vi "CREATE CHECK IN QUERY.vi"(0 "What to Search":string, 5 "Search Column Name":string, 7 "Sorting Column Name":string, 9 "Column to Search In":u16, 11 "Column to Sort By":u16, 12 "Date Range":u16(ring) items=["Greater Than", "Less Than", "Between"], 13 "Dates Less Than":string="8/1/2023", 14 "Dates Greater Than":string="8/1/2023") -> (4 "SQL QUERY":string)   [LabVIEW 2019]
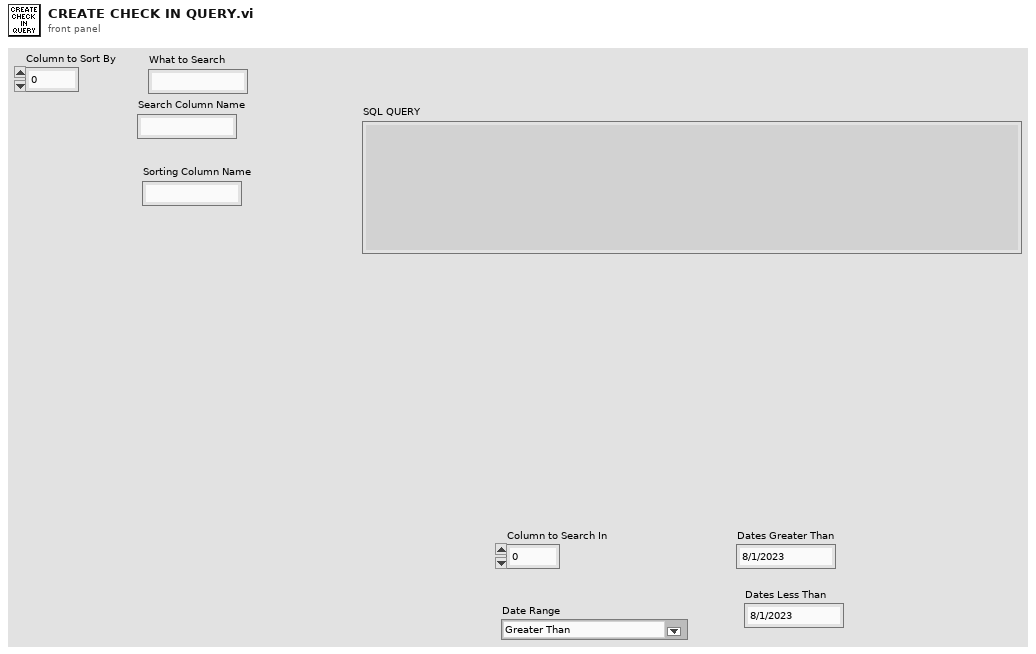
[diagram p1: front panel]
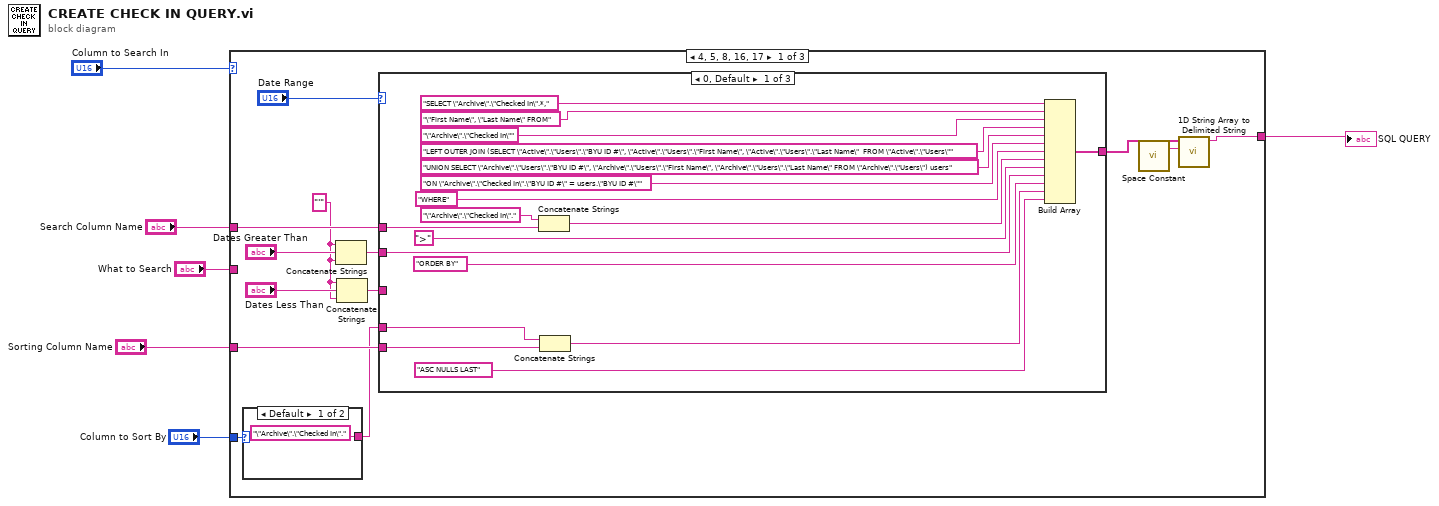
[diagram p0: block diagram]
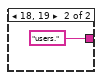
[diagram p2: hidden frame]
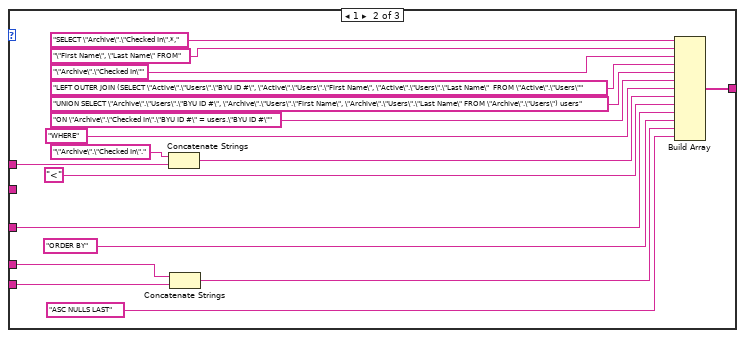
[diagram p3: hidden frame]
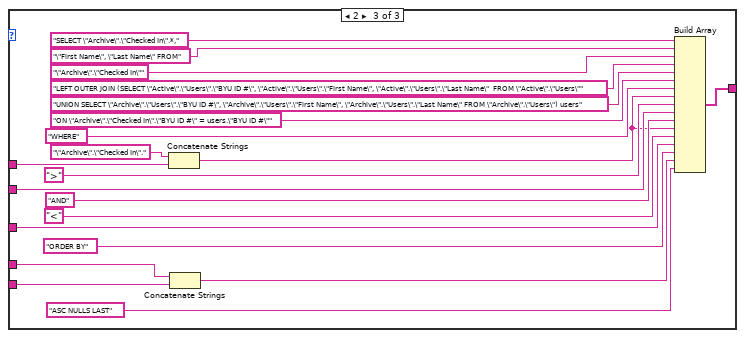
[diagram p4: hidden frame]
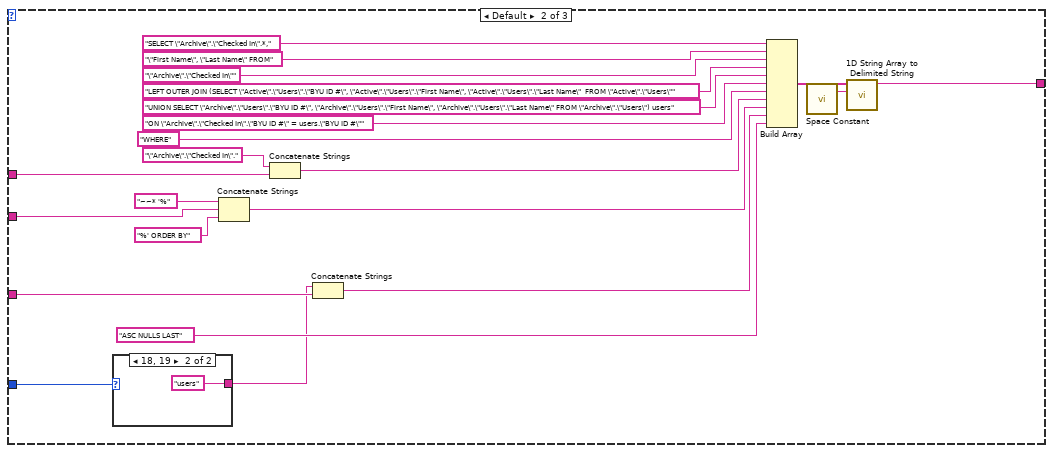
[diagram p5: hidden frame]
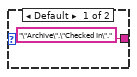
[diagram p6: hidden frame]
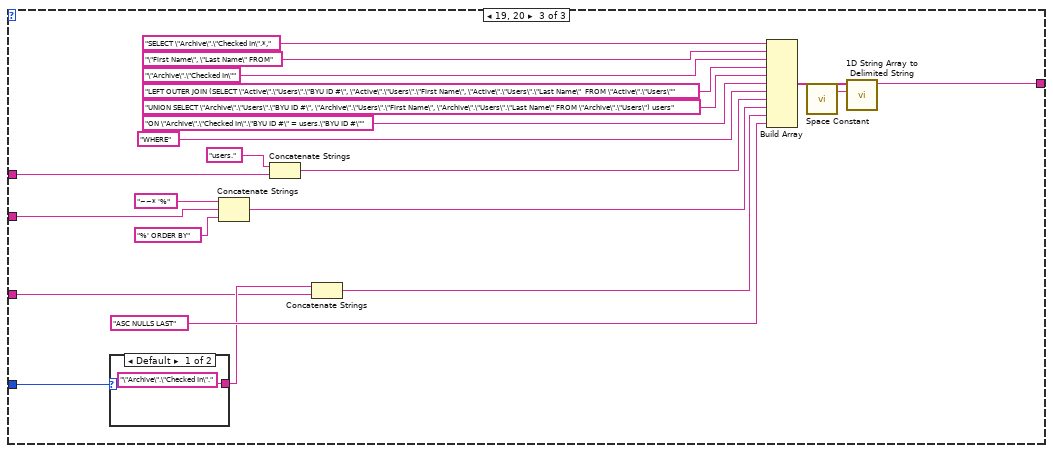
[diagram p7: hidden frame]
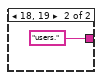
[diagram p8: hidden frame]
diagram:
  n1 = case shown="4, 5, 8, 16, 17" "Column to Search In" {
    tunnel: [w15 w88 w112] -> w6
    tunnel: "Sorting Column Name" -> [w17 w81 w104]
    tunnel: "Search Column Name" -> [w18 w86 w110]
    tunnel: "Column to Sort By" -> [w8 w82 w106]
    tunnel: "What to Search" -> [_ w83 w107]
    frame 4, 5, 8, 16, 17 {
      w9 = "'"
      n2 = case shown="Default" w8 {
        tunnel: ["\"Archive\".\"Checked In\"." ("string") "users." ("string")] -> w7
        frame Default {
        }
        frame 18, 19 {
        }
      }
      n3 = Concatenate Strings(w9, "Dates Greater Than", w9) -> (w13:string)
      n4 = Concatenate Strings(w9, "Dates Less Than", w9) -> (w12:string)
      n5 = case shown="0, Default" "Date Range" {
        tunnel: w18 -> [w32 w50 w71]
        tunnel: w13 -> [w28 _ w66]
        tunnel: w17 -> [w26 w45 w69]
        tunnel: [w23 w42 w68] -> w14
        tunnel: w12 -> [_ w41 w62]
        tunnel: w7 -> [w22 w40 w58]
        frame 0, Default {
          n6 = Concatenate Strings("\"Archive\".\"Checked In\"." ("string"), w32) -> (w30:string)
          n7 = Concatenate Strings(w22, w26) -> (w25:string)
          n8 = Build Array("SELECT \"Archive\".\"Checked In\".*," ("string"), "\"First Name\", \"Last Name\" FROM" ("string"), "\"Archive\".\"Checked In\"" ("string"), "LEFT OUTER JOIN (SELECT \"Active\".\"Users\".\"BYU ID #\", \"Active\".\"Users\".\"First Name\", \"Active\".\"Users\".\"Last Name\"  FROM \"Active\".\"Users\"" ("string"), "UNION SELECT \"Archive\".\"Users\".\"BYU ID #\", \"Archive\".\"Users\".\"First Name\", \"Archive\".\"Users\".\"Last Name\" FROM \"Archive\".\"Users\") users" ("string"), "ON \"Archive\".\"Checked In\".\"BYU ID #\" = users.\"BYU ID #\"" ("string"), "WHERE" ("string"), w30, ">" ("string"), w28, "ORDER BY" ("string"), w25, "ASC NULLS LAST" ("string")) -> (w23:string[])
        }
        frame 1 {
          n9 = Concatenate Strings("\"Archive\".\"Checked In\"." ("string"), w50) -> (w48:string)
          n10 = Concatenate Strings(w40, w45) -> (w44:string)
          n11 = Build Array("SELECT \"Archive\".\"Checked In\".*," ("string"), "\"First Name\", \"Last Name\" FROM" ("string"), "\"Archive\".\"Checked In\"" ("string"), "LEFT OUTER JOIN (SELECT \"Active\".\"Users\".\"BYU ID #\", \"Active\".\"Users\".\"First Name\", \"Active\".\"Users\".\"Last Name\"  FROM \"Active\".\"Users\"" ("string"), "UNION SELECT \"Archive\".\"Users\".\"BYU ID #\", \"Archive\".\"Users\".\"First Name\", \"Archive\".\"Users\".\"Last Name\" FROM \"Archive\".\"Users\") users" ("string"), "ON \"Archive\".\"Checked In\".\"BYU ID #\" = users.\"BYU ID #\"" ("string"), "WHERE" ("string"), w48, "<" ("string"), w41, "ORDER BY" ("string"), w44, "ASC NULLS LAST" ("string")) -> (w42:string[])
        }
        frame 2 {
          n12 = Concatenate Strings("\"Archive\".\"Checked In\"." ("string"), w71) -> (w64:string)
          n13 = Concatenate Strings(w58, w69) -> (w60:string)
          n14 = Build Array("SELECT \"Archive\".\"Checked In\".*," ("string"), "\"First Name\", \"Last Name\" FROM" ("string"), "\"Archive\".\"Checked In\"" ("string"), "LEFT OUTER JOIN (SELECT \"Active\".\"Users\".\"BYU ID #\", \"Active\".\"Users\".\"First Name\", \"Active\".\"Users\".\"Last Name\"  FROM \"Active\".\"Users\"" ("string"), "UNION SELECT \"Archive\".\"Users\".\"BYU ID #\", \"Archive\".\"Users\".\"First Name\", \"Archive\".\"Users\".\"Last Name\" FROM \"Archive\".\"Users\") users" ("string"), "ON \"Archive\".\"Checked In\".\"BYU ID #\" = users.\"BYU ID #\"" ("string"), "WHERE" ("string"), w64, ">" ("string"), w66, "AND" ("string"), w64, "<" ("string"), w62, "ORDER BY" ("string"), w60, "ASC NULLS LAST" ("string")) -> (w68:string[])
        }
      }
      n15 = call <vilib>:"Space Constant.vi"() -> ("String"=w16:string)
      n16 = call <vilib>:"1D String Array to Delimited String.vi"("delimiter"=w16, "string array"=w14) -> ("delimited string"=w15:string)  [unwired: 9 in]
    }
    frame Default {
      n17 = case shown="18, 19" w82 {
        tunnel: ["\"Archive\".\"Checked In\"." ("string") "users" ("string")] -> w80
        frame Default {
        }
        frame 18, 19 {
        }
      }
      n18 = Concatenate Strings("~~* '%" ("string"), w83, "%' ORDER BY" ("string")) -> (w95:string)
      n19 = Concatenate Strings("\"Archive\".\"Checked In\"." ("string"), w86) -> (w84:string)
      n20 = Concatenate Strings(w80, w81) -> (w79:string)
      n21 = Build Array("SELECT \"Archive\".\"Checked In\".*," ("string"), "\"First Name\", \"Last Name\" FROM" ("string"), "\"Archive\".\"Checked In\"" ("string"), "LEFT OUTER JOIN (SELECT \"Active\".\"Users\".\"BYU ID #\", \"Active\".\"Users\".\"First Name\", \"Active\".\"Users\".\"Last Name\"  FROM \"Active\".\"Users\"" ("string"), "UNION SELECT \"Archive\".\"Users\".\"BYU ID #\", \"Archive\".\"Users\".\"First Name\", \"Archive\".\"Users\".\"Last Name\" FROM \"Archive\".\"Users\") users" ("string"), "ON \"Archive\".\"Checked In\".\"BYU ID #\" = users.\"BYU ID #\"" ("string"), "WHERE" ("string"), w84, w95, w79, "ASC NULLS LAST" ("string")) -> (w99:string[])
      n22 = call <vilib>:"Space Constant.vi"() -> ("String"=w98:string)
      n23 = call <vilib>:"1D String Array to Delimited String.vi"("delimiter"=w98, "string array"=w99) -> ("delimited string"=w88:string)  [unwired: 9 in]
    }
    frame 19, 20 {
      n24 = case shown="Default" w106 {
        tunnel: ["\"Archive\".\"Checked In\"." ("string") "users." ("string")] -> w105
        frame Default {
        }
        frame 18, 19 {
        }
      }
      n25 = Concatenate Strings("~~* '%" ("string"), w107, "%' ORDER BY" ("string")) -> (w119:string)
      n26 = Concatenate Strings("users." ("string"), w110) -> (w108:string)
      n27 = Concatenate Strings(w105, w104) -> (w103:string)
      n28 = Build Array("SELECT \"Archive\".\"Checked In\".*," ("string"), "\"First Name\", \"Last Name\" FROM" ("string"), "\"Archive\".\"Checked In\"" ("string"), "LEFT OUTER JOIN (SELECT \"Active\".\"Users\".\"BYU ID #\", \"Active\".\"Users\".\"First Name\", \"Active\".\"Users\".\"Last Name\"  FROM \"Active\".\"Users\"" ("string"), "UNION SELECT \"Archive\".\"Users\".\"BYU ID #\", \"Archive\".\"Users\".\"First Name\", \"Archive\".\"Users\".\"Last Name\" FROM \"Archive\".\"Users\") users" ("string"), "ON \"Archive\".\"Checked In\".\"BYU ID #\" = users.\"BYU ID #\"" ("string"), "WHERE" ("string"), w108, w119, w103, "ASC NULLS LAST" ("string")) -> (w123:string[])
      n29 = call <vilib>:"Space Constant.vi"() -> ("String"=w122:string)
      n30 = call <vilib>:"1D String Array to Delimited String.vi"("delimiter"=w122, "string array"=w123) -> ("delimited string"=w112:string)  [unwired: 9 in]
    }
  }
  "SQL QUERY" <- w6
